vi "Calculate Plot Range.vi"(8 "error in (no error)":errorcluster, 9 "Coordinates System":enum16{"Cartesian", "Cylindrical", "Spherical"}(ring), 10 "3D Bar Datatype.lvclass in":refnum<class "3D Bar Datatype.lvclass">, 11 "Plot Representation In":T1) -> (0 "error out":errorcluster, 2 "3D Bar Datatype.lvclass out":refnum<class "3D Bar Datatype.lvclass">, 3 "Plot Representation Out":T1)   [LabVIEW 2017, in "3D Bar Datatype.lvclass"]
uses:
  <vilib>/Math Plots/3D Math Plots/3D Bar/3D Bar Datatype/3D Bar Datatype.lvclass
  <vilib>/Math Plots/3D Math Plots/3D Plot/3D Plot/Typedef/Plot Representation.ctl
  <vilib>/Math Plots/3D Math Plots/3D Plot/3D Plot/Typedef/Range Clusters.ctl
  <vilib>/Math Plots/3D Math Plots/3D Plot/3D Plot/Typedef/Mesh Data.ctl
  <vilib>/Math Plots/3D Math Plots/3D Bar/3D Bar Datatype/3D Bar Datatype.lvclass/3D Bar Datatype.ctl
  <vilib>/Math Plots/3D Math Plots/3D Plot/3D Plot/3D Plot.lvclass
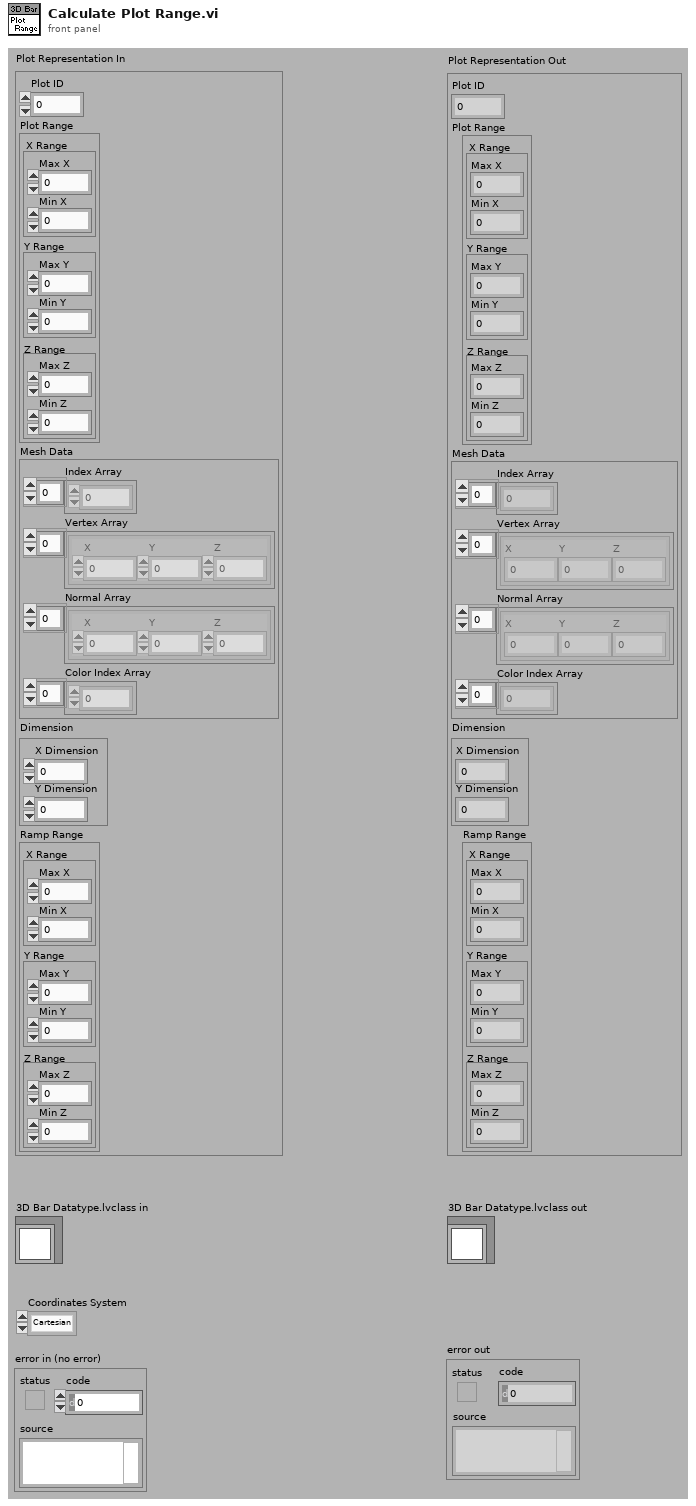
[diagram p1: front panel]
types:
  T1 = typedef "3D Plot.lvclass/Plot Representation.ctl" = cluster{"Plot ID":i32, "Plot Range":T2, "Mesh Data":T3, "Dimension":cluster{"X Dimension":i32, "Y Dimension":i32}, "Ramp Range":T2}
  T2 = typedef "3D Plot.lvclass/Range Clusters.ctl" = cluster{"X Range":cluster{"Max X":sgl, "Min X":sgl}, "Y Range":cluster{"Max Y":sgl, "Min Y":sgl}, "Z Range":cluster{"Max Z":sgl, "Min Z":sgl}}
  T3 = typedef "3D Plot.lvclass/Mesh Data.ctl" = cluster{"Index Array":u32[], "Vertex Array":cluster{"X":sgl, "Y":sgl, "Z":sgl}[], "Normal Array":cluster{"X":sgl, "Y":sgl, "Z":sgl}[], "Color Index Array":i32[]}
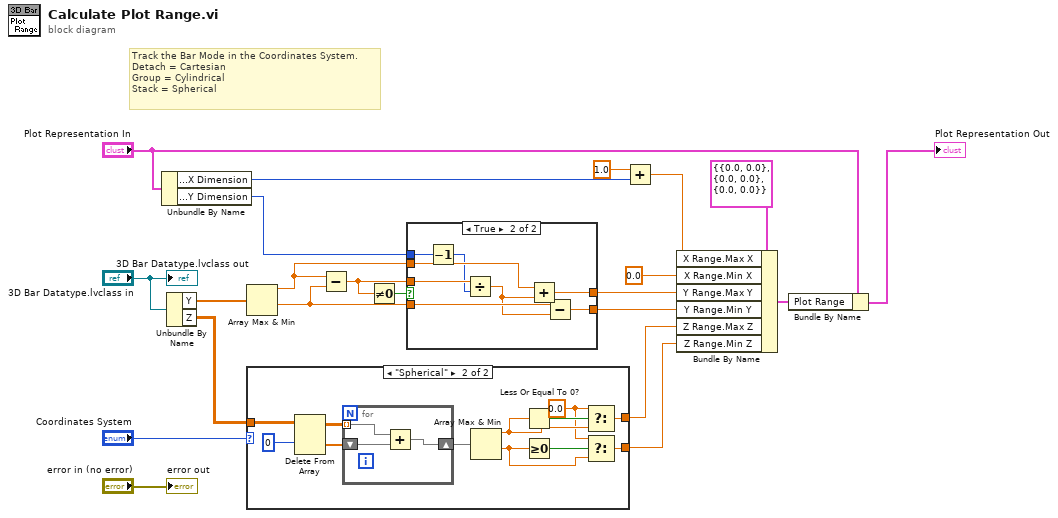
[diagram p0: block diagram]
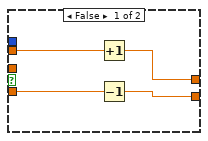
[diagram p2: hidden frame]
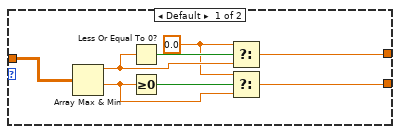
[diagram p3: hidden frame]
diagram:
  # "Track the Bar Mode in the Coordinates System.\nDetach = Cartesian\nGroup = Cylindrical\nStack = Spherical"
  n1 = Unbundle By Name("Plot Representation In") -> ("Dimension.X Dimension"=w9:i32, "Dimension.Y Dimension"=w1:i32)
  n2 = Unbundle By Name("3D Bar Datatype.lvclass in") -> ("Y"=w6:sgl[], "Z"=w13:sgl[][])
  n3 = Array Max & Min(array=w6) -> (max value=w5:sgl, min value=w4:sgl)  [unwired: 2 out]
  n4 = case shown="\"Spherical\"" "Coordinates System" {
    tunnel: [w25 w31] -> w15
    tunnel: [w24 w32] -> w14
    tunnel: w13 -> [w23 w41]
    frame Default {
      w27 = sgl 0.0 ("t")
      n5 = Array Max & Min(array=w23) -> (max value=w28:sgl, min value=w26:sgl)  [unwired: 2 out]
      n6 = Less Or Equal To 0?(x=w28) -> (x <= 0?=w30:bool)
      n7 = Greater Or Equal To 0?(x=w26) -> (x >= 0?=w29:bool)
      n8 = Select(t=w27, s=w30, f=w28) -> (s? t:f=w24:sgl)
      n9 = Select(t=w27, s=w29, f=w26) -> (s? t:f=w25:sgl)
    }
    frame "Spherical" {
      w35 = sgl 0.0 ("t")
      n10 = Delete From Array(array=w41, index (row)=0) -> (deleted portion=w39:sgl[], array with subset deleted=w42:sgl[][])  [unwired: 2 in]
      n11 = for {
        tunnel: w42 -> [w45] mode=indexing
        shift-right: [w43] -> w33
        shift-left: w39 -> [w44]
        n12 = Add(x=w45, y=w44) -> (x+y=w43:sgl[])
      }
      n13 = Array Max & Min(array=w33) -> (max value=w36:sgl, min value=w34:sgl)  [unwired: 2 out]
      n14 = Less Or Equal To 0?(x=w36) -> (x <= 0?=w38:bool)
      n15 = Greater Or Equal To 0?(x=w34) -> (x >= 0?=w37:bool)
      n16 = Select(t=w35, s=w38, f=w36) -> (s? t:f=w32:sgl)
      n17 = Select(t=w35, s=w37, f=w34) -> (s? t:f=w31:sgl)
    }
  }
  n18 = Subtract(x=w5, y=w4) -> (x-y=w2:sgl)
  n19 = Not Equal To 0?(x=w2) -> (x != 0?=w3:bool)
  n20 = case shown="True" w3 {
    tunnel: [w48 w57] -> w8
    tunnel: [w46 w56] -> w7
    tunnel: w5 -> [w49 w55]
    tunnel: w4 -> [w47 w54]
    tunnel: w1 -> [_ w52]
    tunnel: w2 -> [_ w51]
    frame False {
      n21 = Increment(x=w49) -> (x+1=w48:sgl)
      n22 = Decrement(x=w47) -> (x-1=w46:sgl)
    }
    frame True {
      n23 = Decrement(x=w52) -> (x-1=w50:i32)
      n24 = Divide(x=w51, y=w50) -> (x/y=w53:sgl)
      n25 = Add(x=w55, y=w53) -> (x+y=w57:sgl)
      n26 = Subtract(x=w54, y=w53) -> (x-y=w56:sgl)
    }
  }
  n27 = Add(x=sgl 1.0 ("X Range.Min"), y=w9) -> (x+y=w10:sgl)
  n28 = Bundle By Name(cluster=T2 {"X Range"={"Max X"=0.0, "Min X"=0.0}, "Y Range"={"Max Y"=0.0, "Min Y"=0.0}, "Z Range"={"Max Z"=0.0, "Min Z"=0.0}} ("This Range Min/Max Out"), "X Range.Max X"=w10, "X Range.Min X"=sgl 0.0 ("X Range.Min"), "Y Range.Max Y"=w8, "Y Range.Min Y"=w7, "Z Range.Max Z"=w14, "Z Range.Min Z"=w15) -> (w16:T2)
  n29 = Bundle By Name(cluster="Plot Representation In", "Plot Range"=w16) -> (→"Plot Representation Out":T1)
  "error out" <- "error in (no error)"
  "3D Bar Datatype.lvclass out" <- "3D Bar Datatype.lvclass in"
